vi "Tree_Filter_2 Maintain Heirarchy.vi"(10 "Filter keeps":bool[](array[boolean]), 11 "Full Tree Array":T1(array[cluster])) -> (1 "Incices removed":i32[](array[numeric]), 2 "Retained Items":bool[](array[boolean]), 3 "Tree Array out":T1(array[cluster]))   [LabVIEW 2023]
doc: "input a tree array and a boolean array of items that pass a prior filtering step. This VI will return an indent-mainteained tree array, apoplying the filter and retaining any parent items required to maintin the indent heirarchy of the tree.\n\nThe Retained Items boolean array output indicates the items that didn't pass the prior filter test but were retained to maintain the tree heirarchy. It is useful to apply this array to disable those retained items in the tree."
panel:
  out "Has kept decendants":bool[](array[boolean])
  out "Decendant Indicies":cluster{"Array":i32[]}[](array[cluster])
  # "for each tree item, get its decendants index and legnth"
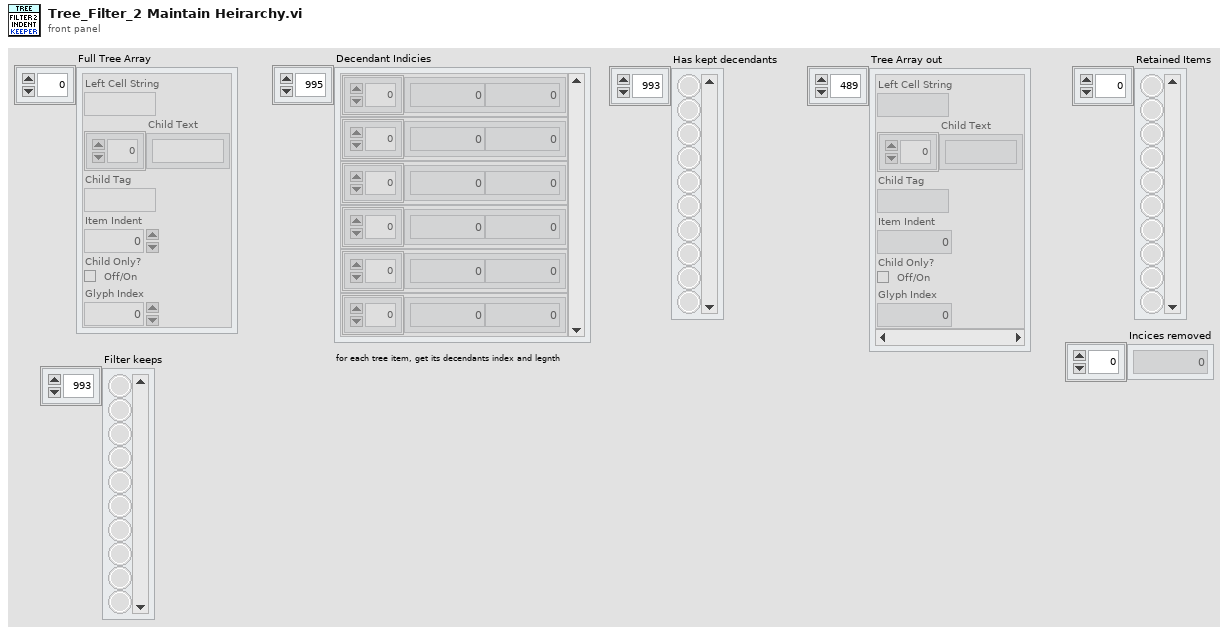
[diagram p1: front panel]
types:
  T1 = cluster{"Left Cell String":string, "Child Text":string[], "Child Tag":string, "Item Indent":i32, "Child Only?":bool, "Glyph Index":i32}[]
  T2 = cluster{"Left Cell String":string, "Child Text":string[], "Child Tag":string, "Item Indent":i32, "Child Only?":bool, "Glyph Index":i32}
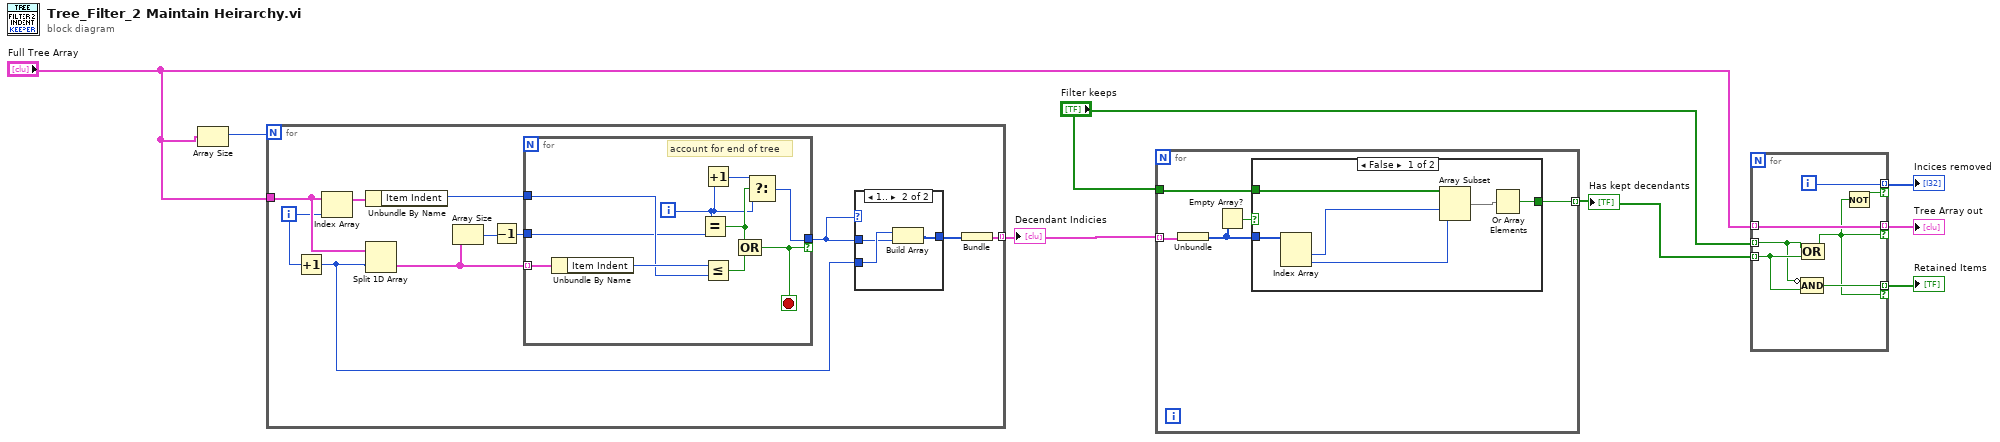
[diagram p0: block diagram]
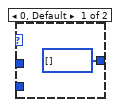
[diagram p2: hidden frame]
diagram:
  n1 = Array Size(array="Full Tree Array") -> (size(s)=w2:i32)
  n2 = for {
    N: w2 -> [_]
    tunnel: "Full Tree Array" -> [w18]
    tunnel: [w14] -> w3 mode=indexing
    i -> [w16]
    n3 = Increment(x=w16) -> (x+1=w13:i32)
    n4 = Index Array(array=w18, index=w16) -> (element=w19:T2)
    n5 = Unbundle By Name(w19) -> ("Item Indent"=w17:i32)
    n6 = Split 1D Array(array=w18, index=w13) -> (second subarray=w11:T1)  [unwired: 1 out]
    n7 = Array Size(array=w11) -> (size(s)=w10:i32)
    n8 = Decrement(x=w10) -> (x-1=w9:i32)
    n9 = for {
      tunnel: w11 -> [w29] mode=indexing
      tunnel: w17 -> [w27]
      tunnel: [w20] -> w12 if=w24
      tunnel: w9 -> [w26]
      i -> [w21]
      stop <- w24 stop-if-true
      # "account for end of tree"
      n10 = Unbundle By Name(w29) -> ("Item Indent"=w28:i32)
      n11 = Equal?(x=w21, y=w26) -> (x = y?=w22:bool)
      n12 = Increment(x=w21) -> (x+1=w23:i32)
      n13 = Less Or Equal?(x=w28, y=w27) -> (x <= y?=w25:bool)
      n14 = Compound Arithmetic op=OR(w22, w25) -> (w24:bool)
      n15 = Select(t=w23, s=w22, f=w21) -> (s? t:f=w20:i32)
    }
    n16 = case shown="1.." w12 {
      tunnel: [i32[] [] w33] -> w15
      tunnel: w13 -> [_ w32]
      tunnel: w12 -> [_ w31]
      frame 0, Default {
      }
      frame 1.. {
        n17 = Build Array(w32, w31) -> (w33:i32[])
      }
    }
    n18 = Bundle(w15) -> (w14:cluster{i32[]})  [unwired: 1 in]
  }
  "Decendant Indicies" <- w3
  n19 = for {
    tunnel: "Filter keeps" -> [w37]
    tunnel: w3 -> [w38] mode=indexing
    tunnel: [w36] -> w4 mode=indexing
    n20 = Unbundle(w38) -> (w35:i32[])
    n21 = Empty Array?(array=w35) -> (empty?=w34:bool)
    n22 = case shown="False" w34 {
      tunnel: w37 -> [w44 _]
      tunnel: w35 -> [w43 _]
      tunnel: [w41 _] -> w36
      frame False {
        n23 = Index Array(array=w43) -> (element #1=w40:i32, element #2=w39:i32)  [unwired: 2 in]
        n24 = Array Subset(array=w44, index=w40, length=w39) -> (w42:bool[])
        n25 = Or Array Elements(Boolean array=w42) -> (logical OR=w41:bool)
      }
      frame True {
      }
    }
  }
  "Has kept decendants" <- w4
  n26 = for {
    tunnel: "Full Tree Array" -> [w51] mode=indexing
    tunnel: w4 -> [w50] mode=indexing
    tunnel: "Filter keeps" -> [w49] mode=indexing
    tunnel: [w51] -> w7 mode=indexing if=w46
    tunnel: [w48] -> w8 mode=indexing if=w46
    tunnel: [w47] -> w1 mode=indexing if=w45
    i -> [w47]
    n27 = Compound Arithmetic op=AND(invert w49, w50) -> (w48:bool)
    n28 = Compound Arithmetic op=OR(w49, w50) -> (w46:bool)
    n29 = Not(x=w46) -> (.not. x?=w45:bool)
  }
  "Retained Items" <- w8
  "Tree Array out" <- w7
  "Incices removed" <- w1
